vi "event_structure2.vi"() -> ()   [LabVIEW 2019]
panel:
  out "XY Graph":cluster{dbl[], dbl[]}(graph)
  in  "stop":bool
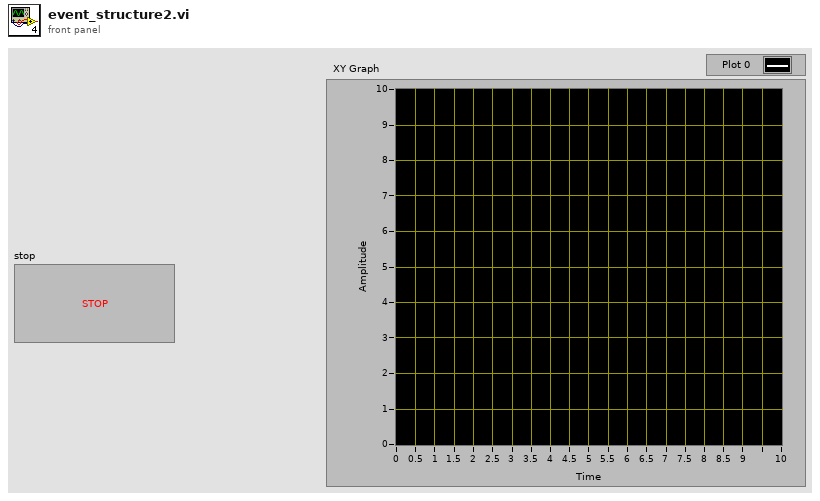
[diagram p1: front panel]
types:
  T1 = typedef "LVPoint32TypeDef.ctl" = cluster{"Horizontal":i32, "Vertical":i32}
  T2 = typedef "LVRectTypeDef.ctl" = cluster{"Left":i16, "Top":i16, "Right":i16, "Bottom":i16}
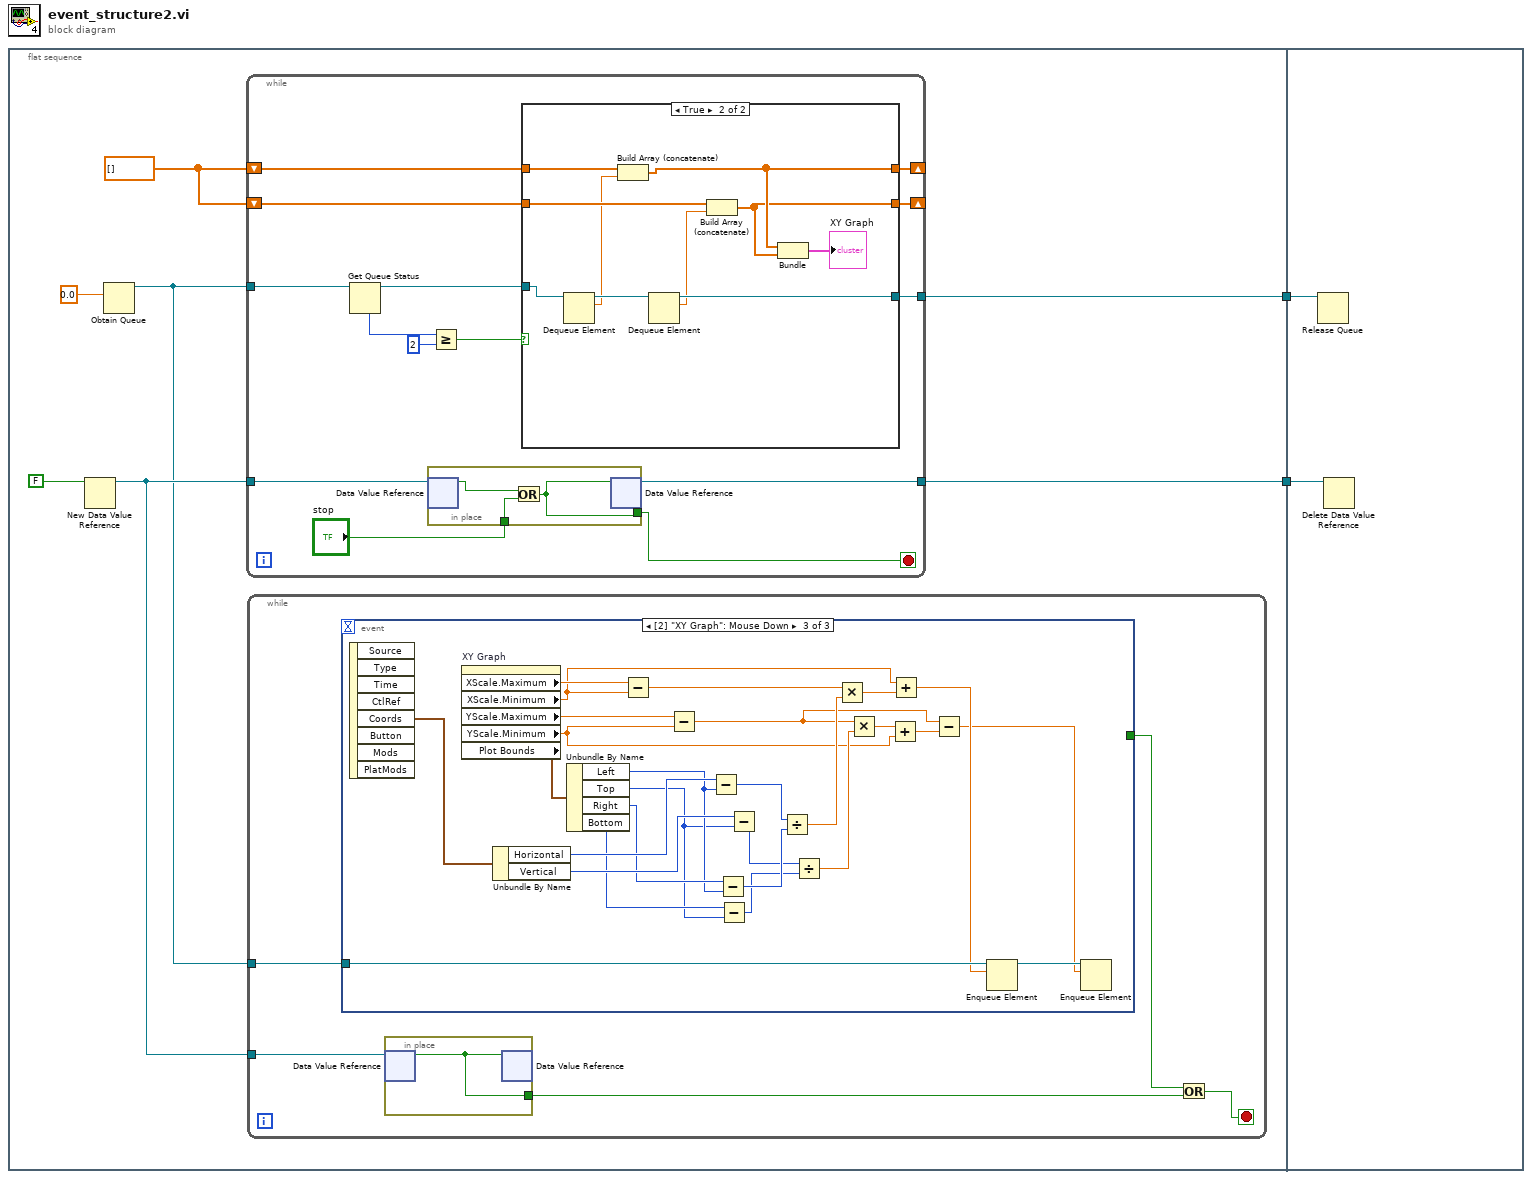
[diagram p0: block diagram]
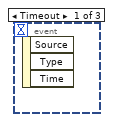
[diagram p3: hidden frame]
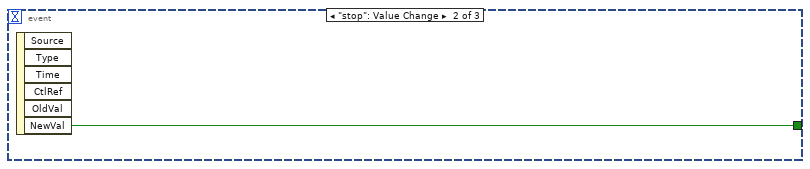
[diagram p4: hidden frame]
diagram:
  n1 = flat-sequence {
    tunnel: [w7] -> w2
    tunnel: [w5] -> w1
    tunnel: w2 -> [w74]
    tunnel: w1 -> [w75]
    frame #0 {
      w4 = dbl[] []
      n2 = New Data Value Reference(data value=FALSE) -> (data value reference=w8:refnum<data-value>)  [unwired: 1 in, 1 out]
      n3 = Obtain Queue(element data type=0.0) -> (queue out=w6:refnum<queue>)  [unwired: 4 in, 2 out]
      n4 = while {
        tunnel: w8 -> [w23]
        tunnel: [w21] -> w7
        tunnel: w6 -> [w19]
        tunnel: [w17] -> w5
        shift-right: [w10] -> _
        shift-left: w4 -> [w13]
        shift-right: [w11] -> _
        shift-left: w4 -> [w12]
        stop <- w20 stop-if-true
        n5 = Get Queue Status(queue=w19) -> (queue out=w18:refnum<queue>, # elements in queue=w16:i32)  [unwired: 2 in, 6 out]
        n6 = in-place {
          in-place-border: "stop" -> [w38]
          in-place-border: [w37] -> w20
          n7 = in-place-dvr #1(w23) -> (w39:bool)  [unwired: 1 out]
          n8 = Or(x=w39, y=w38) -> (x .or. y?=w37:bool)
          n9 = in-place-dvr #1(w37) -> (w21:refnum<data-value>)  [unwired: 1 out]
        }
        n10 = Greater Or Equal?(x=w16, y=2) -> (x >= y?=w15:bool)
        n11 = case shown="True" w15 {
          tunnel: w18 -> [w26 w36]
          tunnel: [w26 w34] -> w17
          tunnel: w13 -> [w25 w33]
          tunnel: w12 -> [w24 w32]
          tunnel: [w24 w28] -> w11
          tunnel: [w25 w29] -> w10
          frame False {
          }
          frame True {
            n12 = Dequeue Element(queue=w36) -> (queue out=w35:refnum<queue>, element=w31:dbl)  [unwired: 2 in, 2 out]
            n13 = Build Array (concatenate)(w33, w31) -> (w29:dbl[])
            n14 = Dequeue Element(queue=w35) -> (queue out=w34:refnum<queue>, element=w30:dbl)  [unwired: 2 in, 2 out]
            n15 = Build Array (concatenate)(w32, w30) -> (w28:dbl[])
            n16 = Bundle(w29, w28) -> (→"XY Graph":cluster{dbl[], dbl[]})  [unwired: 1 in]
          }
        }
      }
      n17 = while {
        tunnel: w8 -> [w44]
        tunnel: w6 -> [w43]
        stop <- w40 stop-if-true
        n18 = event shown="[2] \"XY Graph\": Mouse Down" {
          selector: _ -> [_ _ _]
          dyn-events: _ -> [_ _ _]
          timeout: _ -> [_ _ _]
          tunnel: w43 -> [_ _ w72]
          tunnel: [_ w46 _] -> w42
          event Timeout {
            n19 = event-data() -> ()  [unwired: 1 in, 3 out]
          }
          event "stop": Value Change {
            n20 = event-data() -> ("NewVal"=w46:bool)  [unwired: 1 in, 5 out]
          }
          event "XY Graph": Mouse Down {
            n21 = event-data() -> ("Coords"=w73:T1)  [unwired: 1 in, 7 out]
            n22 = property on="XY Graph" class="XYGraph (strict)"() -> ("XScale.Maximum"=w67:dbl, "XScale.Minimum"=w53:dbl, "YScale.Maximum"=w66:dbl, "YScale.Minimum"=w51:dbl, "Plot Bounds"=w70:T2)  [unwired: 2 in, 2 out]
            n23 = Unbundle By Name(w73) -> ("Horizontal"=w69:i32, "Vertical"=w68:i32)
            n24 = Unbundle By Name(w70) -> ("Left"=w64:i16, "Top"=w62:i16, "Right"=w65:i16, "Bottom"=w63:i16)
            n25 = Subtract(x=w67, y=w53) -> (x-y=w57:dbl)
            n26 = Subtract(x=w66, y=w51) -> (x-y=w49:dbl)
            n27 = Subtract(x=w69, y=w64) -> (x-y=w61:i32)
            n28 = Subtract(x=w65, y=w64) -> (x-y=w60:i16)
            n29 = Subtract(x=w63, y=w62) -> (x-y=w58:i16)
            n30 = Subtract(x=w68, y=w62) -> (x-y=w59:i32)
            n31 = Divide(x=w61, y=w60) -> (x/y=w56:dbl)
            n32 = Divide(x=w59, y=w58) -> (x/y=w55:dbl)
            n33 = Multiply(x=w57, y=w56) -> (x*y=w54:dbl)
            n34 = Multiply(x=w49, y=w55) -> (x*y=w52:dbl)
            n35 = Add(x=w52, y=w51) -> (x+y=w50:dbl)
            n36 = Add(x=w53, y=w54) -> (x+y=w48:dbl)
            n37 = Subtract(x=w49, y=w50) -> (x-y=w47:dbl)
            n38 = Enqueue Element(queue=w72, element=w48) -> (queue out=w71:refnum<queue>)  [unwired: 2 in, 2 out]
            n39 = Enqueue Element(queue=w71, element=w47) -> ()  [unwired: 2 in, 3 out]
          }
        }
        n40 = in-place {
          in-place-border: [w45] -> w41
          n41 = in-place-dvr #2(w44) -> (w45:bool)  [unwired: 1 out]
          n42 = in-place-dvr #2(w45) -> ()  [unwired: 2 out]
        }
        n43 = Or(x=w42, y=w41) -> (x .or. y?=w40:bool)
      }
    }
    frame #1 {
      n44 = Release Queue(queue=w75) -> ()  [unwired: 2 in, 3 out]
      n45 = Delete Data Value Reference(data value reference=w74) -> ()  [unwired: 1 in, 2 out]
    }
  }
